vi "list - get file names.vi"(5 "extension filter":string="*.dat", 7 "regular expression":string="\\s*([0-9]+_.*?)\\.dat\\s*", 11 "folder path":path) -> (0 "Array":string[](array[string]), 2 "OK":bool)   [LabVIEW 2021]
uses:
  <vilib>/regexp/Match Regular Expression.xnode
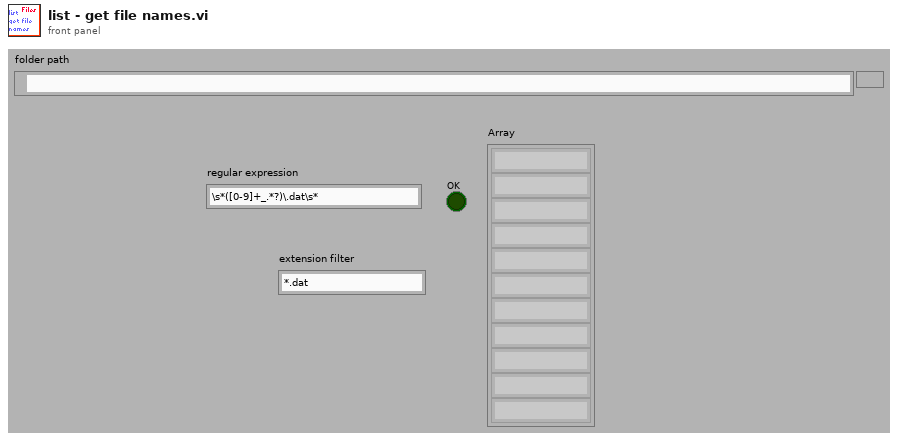
[diagram p1: front panel]
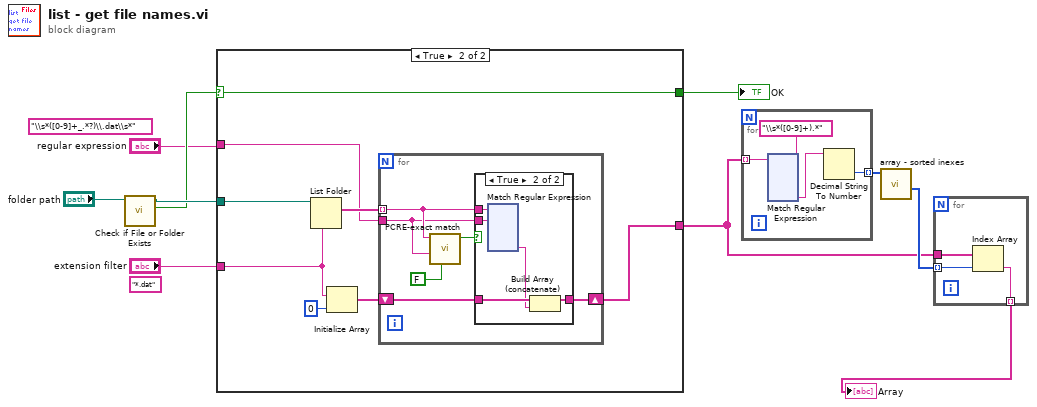
[diagram p0: block diagram]
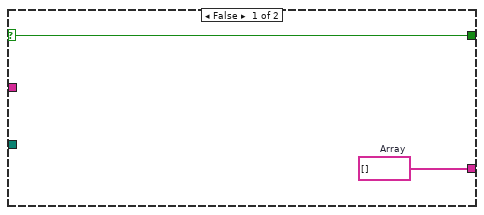
[diagram p2: hidden frame]
diagram:
  (unwired) "\\s*([0-9]+_.*?)\\.dat\\s*" ("regular expression")
  (unwired) "*.dat" ("pattern")
  n1 = call <vilib>:"Check if File or Folder Exists.vi"("path"="folder path") -> ("file or folder exists?"=w8:bool, "dup path"=w9:path)  [unwired: 8 in, 1 out]
  n2 = case shown="True" w8 {
    selector: w8 -> [w11 w13]
    tunnel: "extension filter" -> [_ w19]
    tunnel: "regular expression" -> [_ w16]
    tunnel: w9 -> [_ w15]
    tunnel: [w12 w14] -> w3
    tunnel: [w11 w13] -> w1
    frame False {
      w12 = string[] []  # Array
    }
    frame True {
      n3 = List Folder(path=w15, pattern=w19) -> (filenames=w20:string[])  [unwired: 2 in, 3 out]
      n4 = Initialize Array(w19, 0 ("dimension size")) -> (w17:string[])
      n5 = for {
        tunnel: w20 -> [w24] mode=indexing
        shift-right: [w25] -> w14
        shift-left: w17 -> [w26]
        tunnel: w16 -> [w22]
        n6 = call "PCRE-exact match.vi"("quote specials"=FALSE ("Boolean"), "regular expression"=w22, "input string"=w24) -> ("exact match"=w23:bool)  [unwired: 6 in, 2 out]
        n7 = case shown="True" w23 {
          tunnel: w22 -> [_ w32]
          tunnel: w26 -> [w27 w31]
          tunnel: [w27 w29] -> w25
          tunnel: w24 -> [_ w28]
          frame False {
          }
          frame True {
            n8 = xnode "Match Regular Expression"("input string"=w28, "regular expression"=w32) -> ("submatch 1"=w30:string)  [unwired: 4 in, 5 out]
            n9 = Build Array (concatenate)(w31, w30) -> (w29:string[])
          }
        }
      }
    }
  }
  "OK" <- w1
  n10 = for {
    tunnel: w3 -> [w155] mode=indexing
    tunnel: [w152] -> w5 mode=indexing
    n11 = xnode "Match Regular Expression"("input string"=w155, "regular expression"="\\s*([0-9]+).*") -> ("submatch 1"=w153:string)  [unwired: 4 in, 5 out]
    n12 = Decimal String To Number(string=w153) -> (number=w152:i32)  [unwired: 2 in, 1 out]
  }
  n13 = call "array - sorted inexes.vi"("x"=w5) -> ("index array"=w4:i32[])  [unwired: 9 in, 1 out]
  n14 = for {
    tunnel: w4 -> [w277] mode=indexing
    tunnel: w3 -> [w276]
    tunnel: [w275] -> w2 mode=indexing
    n15 = Index Array(array=w276, index=w277) -> (element=w275:string)
  }
  "Array" <- w2
